vi "F Dwf Enum Config Info.vi"(8 "error in (no error)":errorcluster, 9 "pv":i32, 10 "info":i32, 11 "idxConfig":i32) -> (0 "error out":errorcluster, 1 "pv out":i32, 3 "function return":i32)   [LabVIEW 2019, in "Olasdwf.lvlib"]
doc: "DWFAPI int FDwfEnumConfigInfo(int idxConfig, DwfEnumConfigInfo info, int *pv);"
uses:
  Olasdwf.lvlib
  Windows/System32/dwf.dll
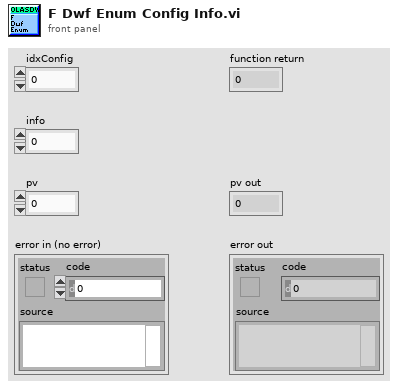
[diagram p1: front panel]
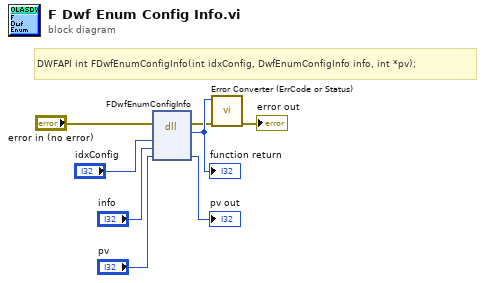
[diagram p0: block diagram]
diagram:
  # "DWFAPI int FDwfEnumConfigInfo(int idxConfig, DwfEnumConfigInfo info, int *pv);"
  n1 = dll-call lib="C:/Windows/System32/dwf.*" fn="FDwfEnumConfigInfo"(error in="error in (no error)", "idxConfig"="idxConfig", "info"="info", "pv"="pv") -> (error out=w2:errorcluster, w8:i32, "pv"=→"pv out":i32)  [unwired: 4 in, 1 out]
  "function return" <- w8
  n2 = call "Error Converter (ErrCode or Status).vi"("error in (no error)"=w2, "error code"=w8) -> ("error out"=→"error out":errorcluster)  [unwired: 9 in]
